vi "顶层容器-网络服务器.vi"() -> ()   [LabVIEW 2013]
panel:
  out "管-监测模式状态？":refnum<vi>
  out "管-停止信号（枚举）":refnum<vi>
  out "管-监测窗口 按钮":refnum<vi>
  in  "监-外部停止信号":refnum<vi>
  out "管理窗口VI-引用":refnum<vi>
  out "管-监测窗口VI-控件引用":refnum<vi>
  in  "管理模式":bool
  in  "监测模式":bool
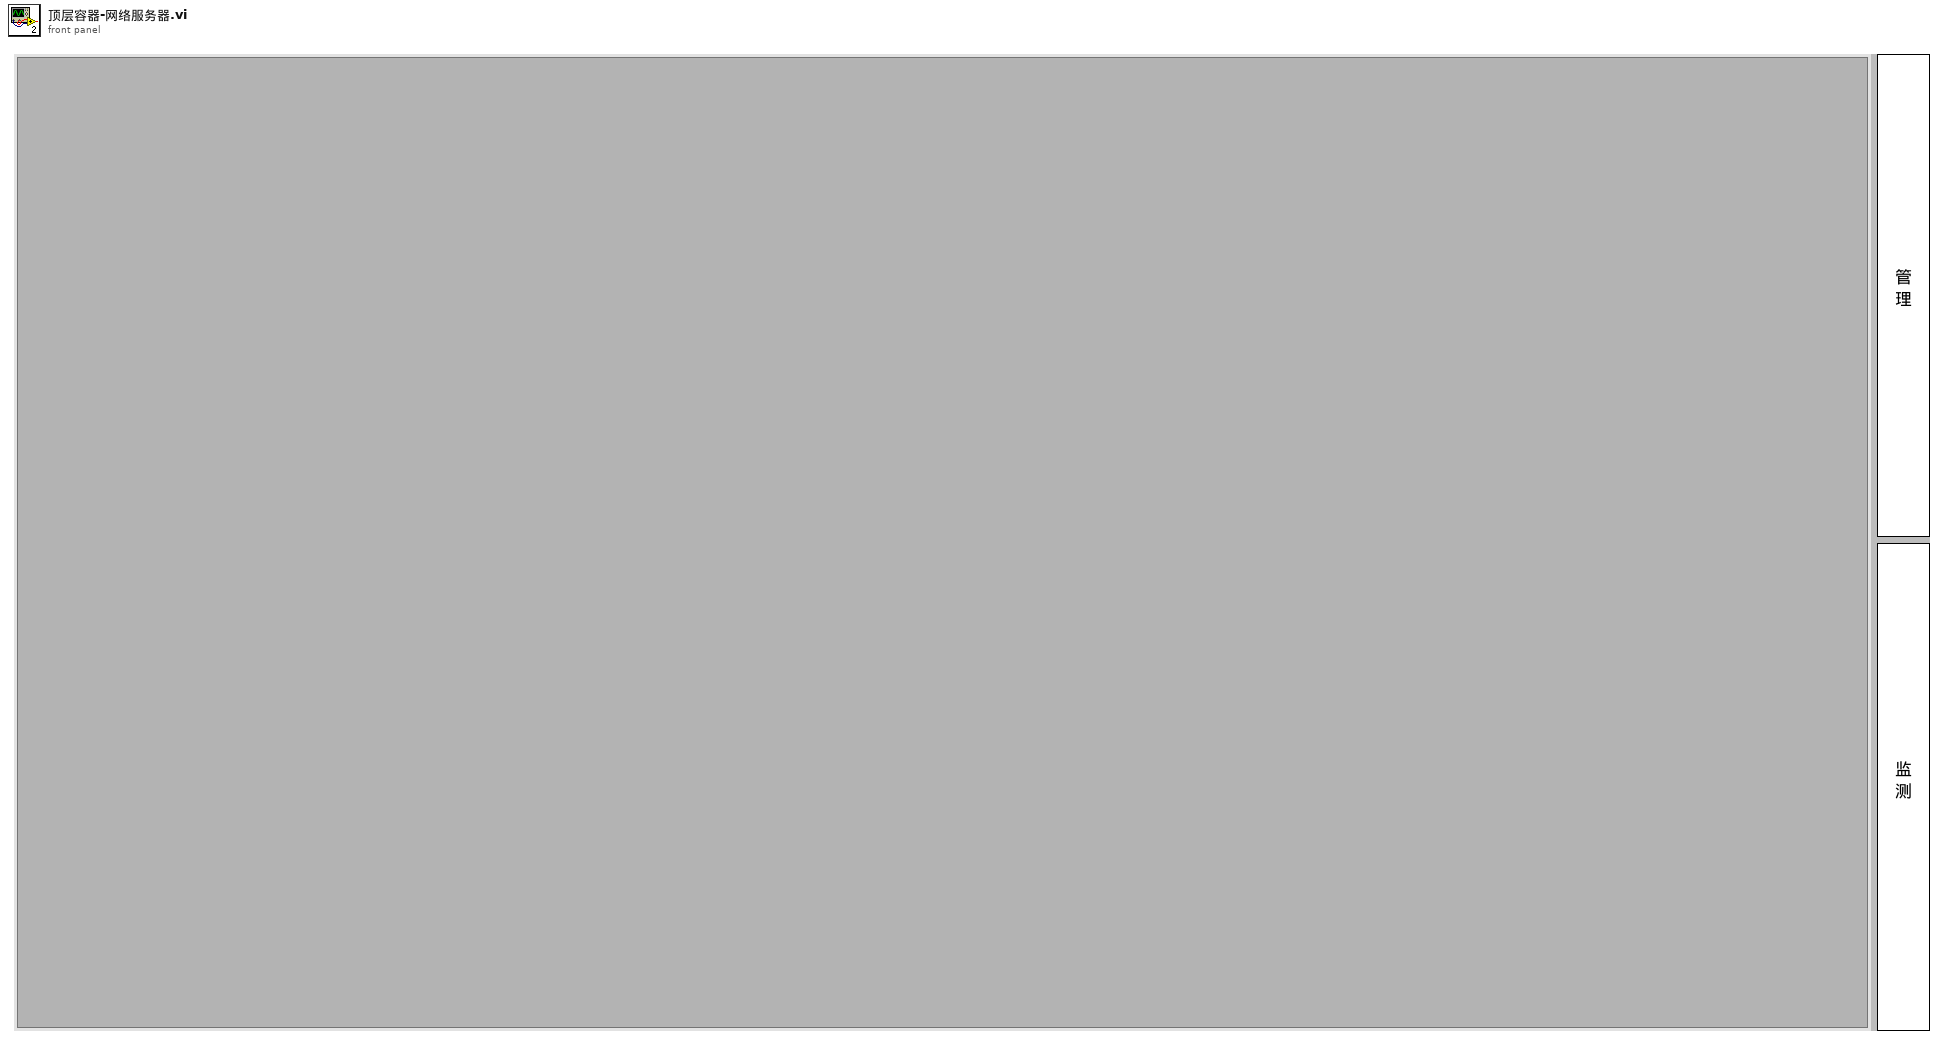
[diagram p1: front panel]
types:
  T1 = enum8{"Enabled", "Disabled", "Disabled and Grayed Out"}
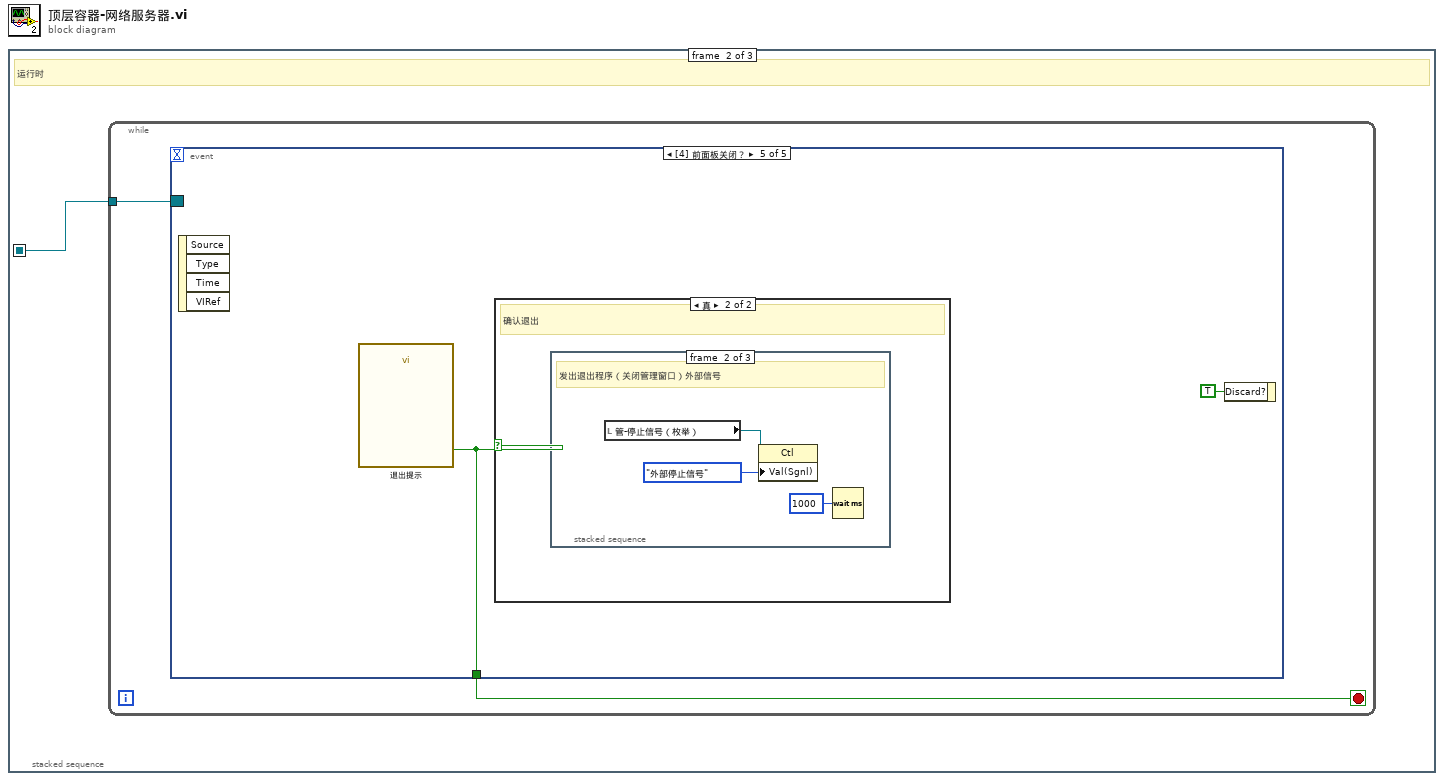
[diagram p0: block diagram]
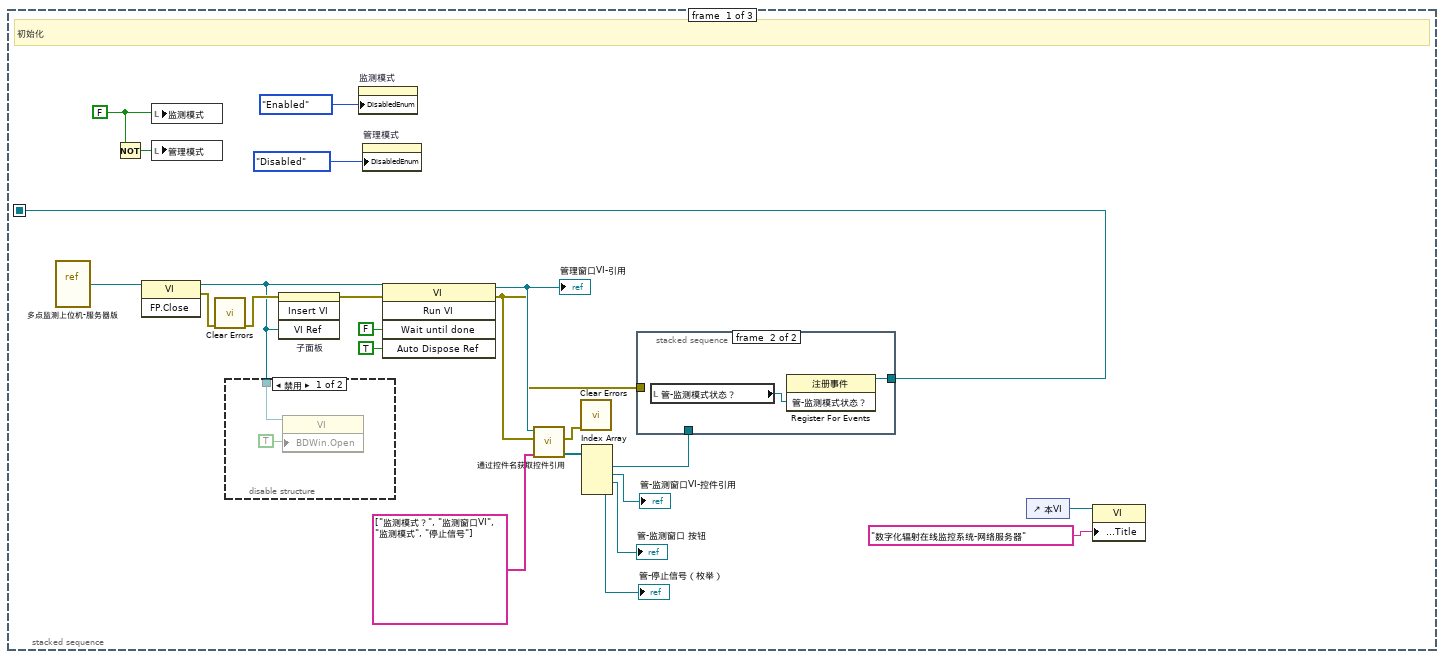
[diagram p2: hidden frame]
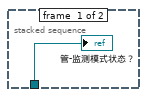
[diagram p4: hidden frame]
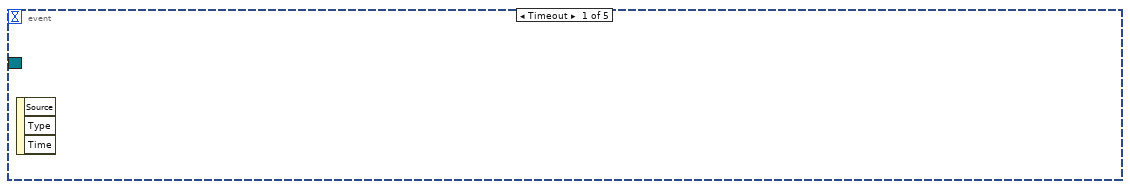
[diagram p5: hidden frame]
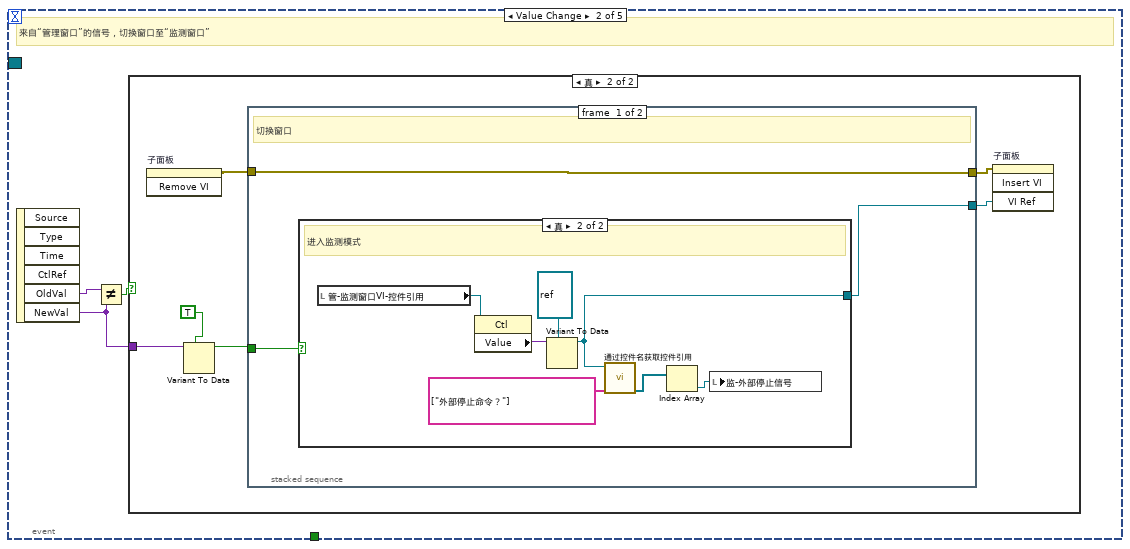
[diagram p6: hidden frame]
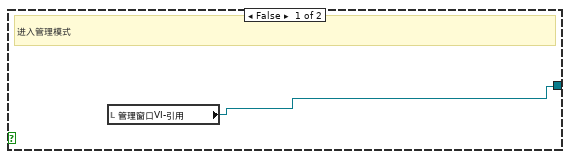
[diagram p8: hidden frame]
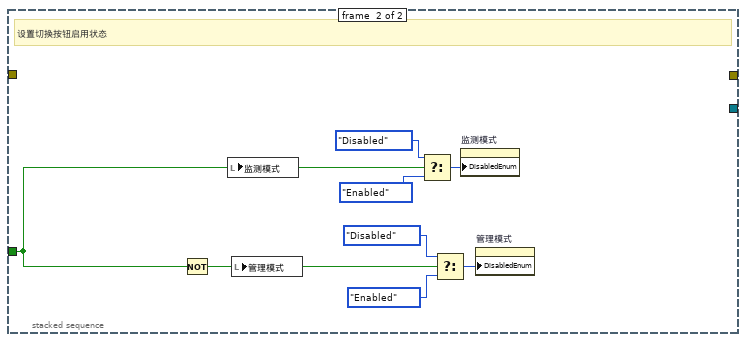
[diagram p9: hidden frame]
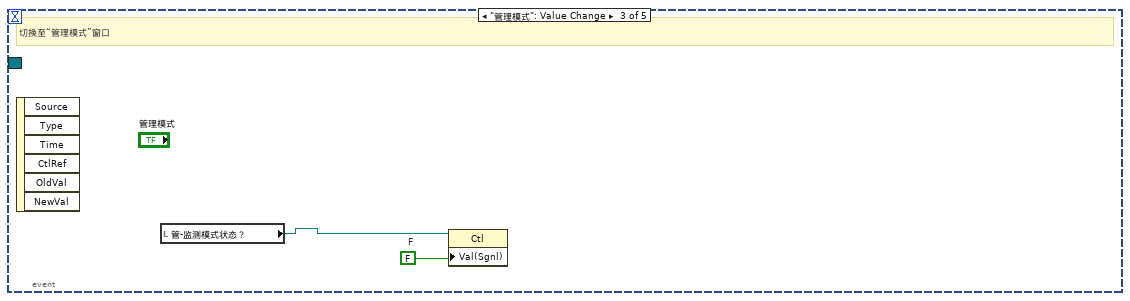
[diagram p10: hidden frame]
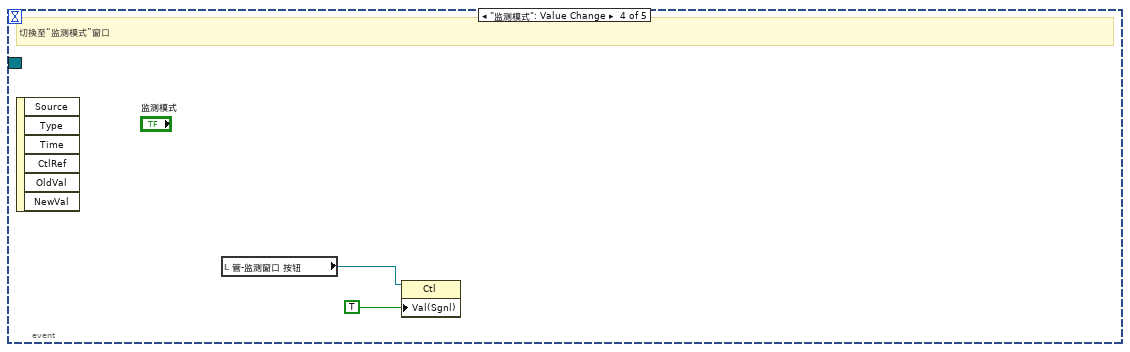
[diagram p11: hidden frame]
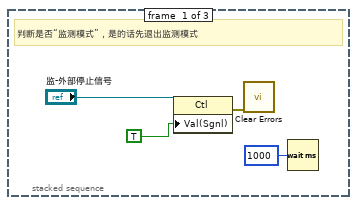
[diagram p13: hidden frame]
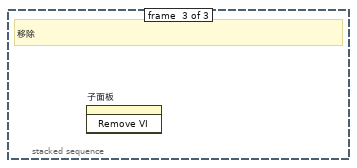
[diagram p14: hidden frame]
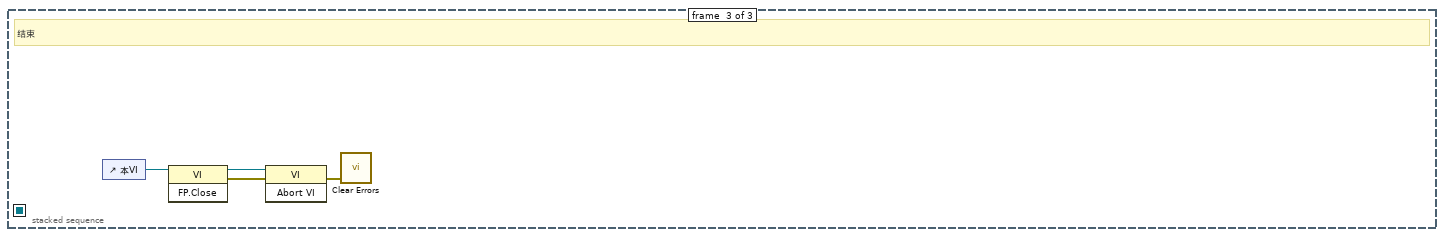
[diagram p15: hidden frame]
diagram:
  n1 = stacked-sequence {
    seq-local: [w16 _ _] -> [_ w29 _]
    frame #0 {
      w23 = FALSE ("监测模式")
      # "初始化"
      n2 = vi-ref "多点监测上位机-服务器版.vi"() -> (w8:refnum<vi>)
      n3 = Not(x=w23) -> (.not. x?=w22:bool)
      n4 = invoke class="VI" method="FP.Close"(reference=w8) -> (reference out=w4:refnum<vi>, error out=w6:errorcluster)  [unwired: 2 in, 1 out]
      n5 = local write "监测模式"(w23) -> ()
      n6 = local write "管理模式"(w22) -> ()
      n7 = call <vilib>:"Clear Errors.vi"("error in (no error)"=w6) -> ("error out"=w5:errorcluster)  [unwired: 6 in]
      n8 = disable-structure shown="禁用" {
        disable-tunnel: w4 -> [w25 _]
        frame Disabled {
          n9 = property class="VI"(reference=w25, "BDWin.Open"=TRUE ("程序框图窗口:打开")) -> ()  [unwired: 1 in, 2 out]
        }
        frame Enabled {
        }
      }
      n10 = invoke on="子面板" class="子面板" method="Insert VI"(error in=w5, "VI Ref"=w4) -> (error out=w2:errorcluster)  [unwired: 2 in, 3 out]
      n11 = property on="监测模式" class="Bool (严格)"("DisabledEnum"=T1."Enabled" ("禁用")) -> ()  [unwired: 2 in, 2 out]
      n12 = property on="管理模式" class="Bool (严格)"("DisabledEnum"=T1."Disabled" ("禁用")) -> ()  [unwired: 2 in, 2 out]
      n13 = invoke class="VI" method="Run VI"(reference=w4, error in=w2, "Wait until done"=FALSE ("结束前等待"), "Auto Dispose Ref"=TRUE ("自动销毁引用")) -> (reference out=w17:refnum<vi>, error out=w3:errorcluster)  [unwired: 1 in, 3 out]
      "管理窗口VI-引用" <- w17
      n14 = call "通过控件名获取控件引用.vi"("控件名数组"=string[] ["监测模式？", "监测窗口VI", "监测模式", "停止信号"], "错误输入（无错误）"=w3, "VI引用"=w17) -> ("控件引用输出"=w19:refnum<vi>[], "错误输出"=w7:errorcluster)  [unwired: 6 in, 1 out]
      n15 = call <vilib>:"Clear Errors.vi"("error in (no error)"=w7) -> ()  [unwired: 6 in, 1 out]
      n16 = Index Array(array=w19) -> (element #1=w1:refnum<vi>, element #2=→"管-监测窗口VI-控件引用":refnum<vi>, element #3=→"管-监测窗口 按钮":refnum<vi>, element #4=→"管-停止信号（枚举）":refnum<vi>)  [unwired: 4 in]
      n17 = stacked-sequence {
        tunnel: [_ w28] -> w16
        tunnel: w3 -> [_ _]
        tunnel: w1 -> [w26 _]
        frame #0 {
          "管-监测模式状态？" <- w26
        }
        frame #1 {
          n18 = local read "管-监测模式状态？"() -> (w27:refnum<vi>)
          n19 = register-events(w27) -> (reference out=w28:refnum<event-registration>)  [unwired: 2 in, 1 out]
        }
      }
      n20 = control-ref of="本VI"() -> (w11:refnum<vi>)
      n21 = property class="VI"(reference=w11, "Front Panel.Title"="数字化辐射在线监控系统-网络服务器" ("前面板窗口:标题")) -> ()  [unwired: 1 in, 2 out]
    }
    frame #1 {
      # "运行时"
      n22 = while {
        tunnel: w29 -> [w30]
        stop <- w31 stop-if-true
        n23 = event shown="[4] 前面板关闭？" {
          selector: w30 -> [_ _ _ _ _]
          dyn-events: _ -> [_ _ _ _ _]
          timeout: _ -> [_ _ _ _ _]
          tunnel: [_ _ _ _ w64] -> w31
          event Timeout {
            n24 = event-data() -> ()  [unwired: 1 in, 3 out]
          }
          event Value Change {
            # "来自“管理窗口”的信号，切换窗口至“监测窗口”"
            n25 = event-data() -> ("OldVal"=w34:variant, "NewVal"=w33:variant)  [unwired: 1 in, 4 out]
            n26 = Not Equal?(x=w34, y=w33) -> (x != y?=w32:bool)
            n27 = case shown="真" w32 {
              tunnel: w33 -> [_ w37]
              frame False {
              }
              frame True {
                n28 = invoke on="子面板" class="子面板" method="Remove VI"() -> (error out=w40:errorcluster)  [unwired: 3 in, 2 out]
                n29 = Variant To Data(type=TRUE, Variant=w37) -> (data=w36:bool)  [unwired: 1 in, 1 out]
                n30 = stacked-sequence {
                  tunnel: w36 -> [w43 w59]
                  tunnel: w40 -> [w41 _]
                  tunnel: [w42 _] -> w39
                  tunnel: [w41 _] -> w38
                  frame #0 {
                    # "切换窗口"
                    n31 = case shown="真" w43 {
                      tunnel: [w44 w45] -> w42
                      frame False {
                        # "进入管理模式"
                        n32 = local read "管理窗口VI-引用"() -> (w44:refnum<vi>)
                      }
                      frame True {
                        # "进入监测模式"
                        n33 = local read "管-监测窗口VI-控件引用"() -> (w51:refnum<vi>)
                        n34 = property class="Ctl"(reference=w51) -> ("Value"=w50:variant)  [unwired: 1 in, 2 out]
                        n35 = Variant To Data(type=refnum<vi> refnum ("本VI"), Variant=w50) -> (data=w45:refnum<vi>)  [unwired: 1 in, 1 out]
                        n36 = call "通过控件名获取控件引用.vi"("控件名数组"=string[] ["外部停止命令？"], "VI引用"=w45) -> ("控件引用输出"=w47:refnum<vi>[])  [unwired: 7 in, 2 out]
                        n37 = Index Array(array=w47) -> (element=w46:refnum<vi>)  [unwired: 1 in]
                        n38 = local write "监-外部停止信号"(w46) -> ()
                      }
                    }
                  }
                  frame #1 {
                    # "设置切换按钮启用状态"
                    n39 = Not(x=w59) -> (.not. x?=w54:bool)
                    n40 = local write "监测模式"(w59) -> ()
                    n41 = local write "管理模式"(w54) -> ()
                    n42 = Select(t=T1."Disabled" ("禁用"), s=w59, f=T1."Enabled" ("禁用")) -> (s? t:f=w53:T1)
                    n43 = Select(t=T1."Disabled" ("禁用"), s=w54, f=T1."Enabled" ("禁用")) -> (s? t:f=w52:T1)
                    n44 = property on="监测模式" class="Bool (严格)"("DisabledEnum"=w53) -> ()  [unwired: 2 in, 2 out]
                    n45 = property on="管理模式" class="Bool (严格)"("DisabledEnum"=w52) -> ()  [unwired: 2 in, 2 out]
                  }
                }
                n46 = invoke on="子面板" class="子面板" method="Insert VI"(error in=w38, "VI Ref"=w39) -> ()  [unwired: 2 in, 4 out]
              }
            }
          }
          event "管理模式": Value Change {
            w61 = FALSE  # F
            # "切换至“管理模式”窗口"
            n47 = event-data() -> ()  [unwired: 1 in, 6 out]
            n48 = local read "管-监测模式状态？"() -> (w60:refnum<vi>)
            n49 = property class="Ctl"(reference=w60, "Val(Sgnl)"=w61) -> ()  [unwired: 1 in, 2 out]
          }
          event "监测模式": Value Change {
            # "切换至“监测模式”窗口"
            n50 = event-data() -> ()  [unwired: 1 in, 6 out]
            n51 = local read "管-监测窗口 按钮"() -> (w63:refnum<vi>)
            n52 = property class="Ctl"(reference=w63, "Val(Sgnl)"=TRUE ("监测模式")) -> ()  [unwired: 1 in, 2 out]
          }
          event Panel Close? {
            n53 = event-data() -> ()  [unwired: 1 in, 4 out]
            n54 = call "退出提示"() -> ("确定"=w64:bool)  [unwired: 10 in, 1 out]
            n55 = case shown="真" w64 {
              frame False {
                # "取消推出"
              }
              frame True {
                # "确认退出"
                n56 = stacked-sequence {
                  frame #0 {
                    # "判断是否“监测模式”，是的话先退出监测模式"
                    n57 = property class="Ctl"(reference="监-外部停止信号", "Val(Sgnl)"=TRUE ("监测模式")) -> (error out=w68:errorcluster)  [unwired: 1 in, 1 out]
                    n58 = call <vilib>:"Clear Errors.vi"("error in (no error)"=w68) -> ()  [unwired: 6 in, 1 out]
                    n59 = Wait (ms)(milliseconds to wait=u32 1000 ("等待时间（毫秒）")) -> ()  [unwired: 1 out]
                  }
                  frame #1 {
                    # "发出退出程序（关闭管理窗口）外部信号"
                    n60 = local read "管-停止信号（枚举）"() -> (w72:refnum<vi>)
                    n61 = property class="Ctl"(reference=w72, "Val(Sgnl)"=enum16{"内部停止信号", "外部停止信号"}."外部停止信号" ("值(信号)")) -> ()  [unwired: 1 in, 2 out]
                    n62 = Wait (ms)(milliseconds to wait=u32 1000 ("等待时间（毫秒）")) -> ()  [unwired: 1 out]
                  }
                  frame #2 {
                    # "移除"
                    n63 = invoke on="子面板" class="子面板" method="Remove VI"() -> ()  [unwired: 3 in, 3 out]
                  }
                }
              }
            }
            n64 = event-data("Discard?"=TRUE ("放弃？")) -> ()  [unwired: 1 in, 1 out]
          }
        }
      }
    }
    frame #2 {
      # "结束"
      n65 = control-ref of="本VI"() -> (w76:refnum<vi>)
      n66 = invoke class="VI" method="FP.Close"(reference=w76) -> (reference out=w75:refnum<vi>, error out=w74:errorcluster)  [unwired: 2 in, 1 out]
      n67 = invoke class="VI" method="Abort VI"(reference=w75, error in=w74) -> (error out=w73:errorcluster)  [unwired: 1 in, 2 out]
      n68 = call <vilib>:"Clear Errors.vi"("error in (no error)"=w73) -> ()  [unwired: 6 in, 1 out]
    }
  }
